vi "Read_Image_Dataset.vi"(4 "Img Width":i32=256, 5 "Norm. Scale":sgl=65535.0, 6 "Img Heigth":i32=256, 7 "Norm. Shift":sgl=65535.0, 8 "error in (no error)":errorcluster, 10 "Annotation file":path, 11 "Image File Paths":path[](array[path])) -> (0 "error out":errorcluster, 3 "Dataset":T1)   [LabVIEW 2020]
uses:
  <vilib>/Ngene/DeepLTK/Toolkit/NN_Data/API/DataSet_Types/NN_DataSet(In3D_Out1D).ctl
  <vilib>/Ngene/DeepLTK/Toolkit/NN_Data/API/DataRef_Types/NN_Data_ref(4D_SGL).ctl
  <vilib>/Ngene/DeepLTK/Toolkit/NN_Data/API/DataRef_Types/NN_Data_ref(2D_SGL).ctl
  <vilib>/Ngene/DeepLTK/Toolkit/NN_Data/Controls/NN_Dims(C,H,W).ctl
  <vilib>/Utility/file.llb/Read Delimited Spreadsheet (string).vi
  <vilib>/vision/NI_Vision_Development_Module.lvlib
  <vilib>/Ngene/DeepLTK/Toolkit/Deep_Learning_Toolkit_by_Ngene.lvlib
panel:
  out "Image Type":T5 items=["Grayscale (U8)", "Grayscale (I16)", "Grayscale (SGL)", "Complex (CSG)", "RGB (U32)", "HSL (U32)", "RGB (U64)", "Grayscale (U16)"]
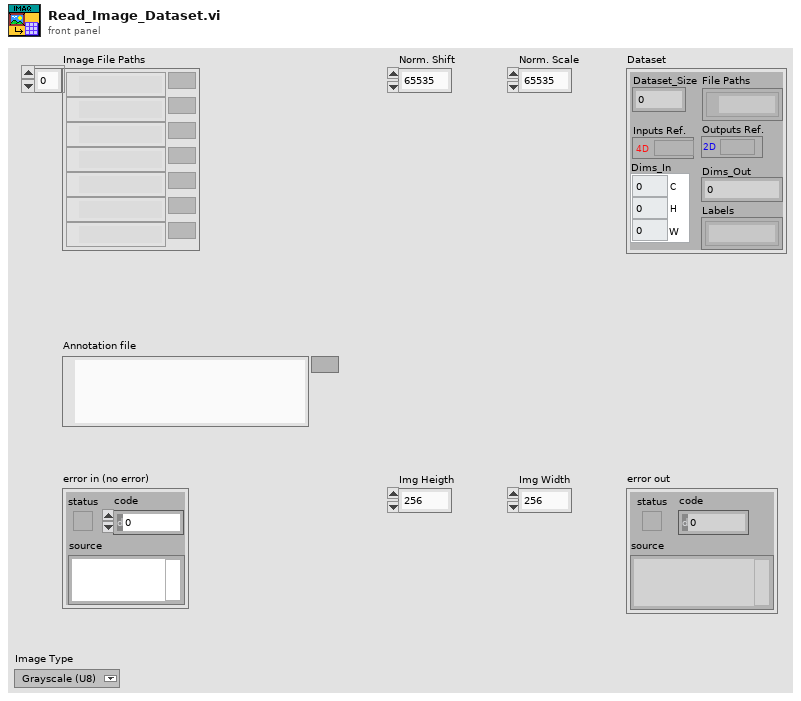
[diagram p1: front panel]
types:
  T1 = typedef "Deep_Learning_Toolkit_by_Ngene.lvlib/NN_DataSet(In3D_Out1D).ctl" = cluster{"Inputs Ref.":T2, "Outputs Ref.":T3, "Dataset_Size":i32, "Dims_In":T4, "Dims_Out":i32, "Labels":string[], "File Paths":path[]}
  T2 = typedef "Deep_Learning_Toolkit_by_Ngene.lvlib/NN_Data_ref(4D_SGL).ctl" = refnum<data-value>
  T3 = typedef "Deep_Learning_Toolkit_by_Ngene.lvlib/NN_Data_ref(2D_SGL).ctl" = refnum<data-value>
  T4 = typedef "Deep_Learning_Toolkit_by_Ngene.lvlib/NN_Dims(C,H,W).ctl" = cluster{"C":i32, "H":i32, "W":i32}
  T5 = typedef "Image Type" = u32
  T6 = typedef "IMAQ Image.ctl" = refnum<image>
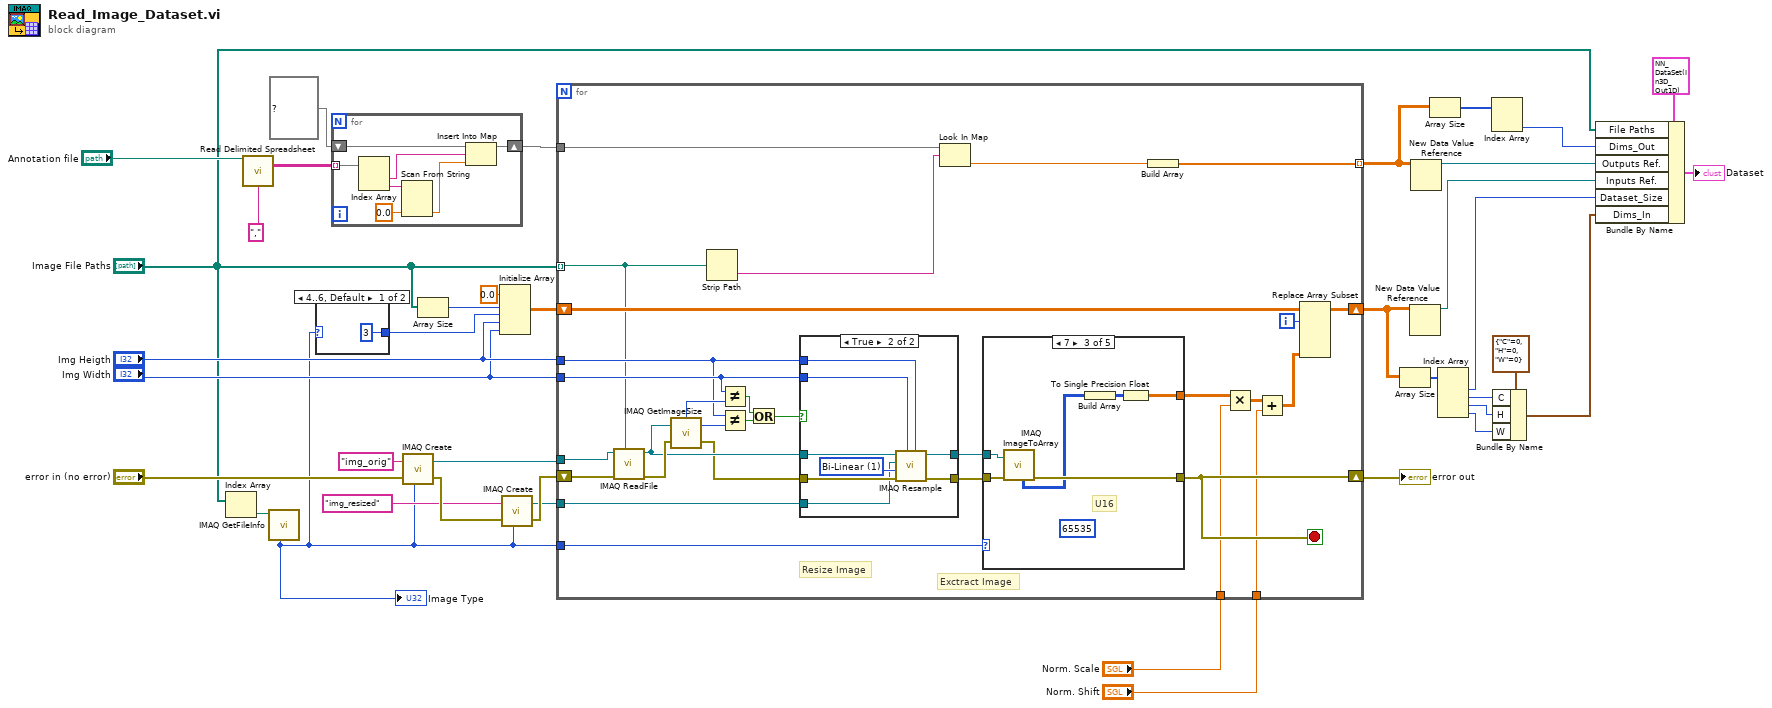
[diagram p0: block diagram]
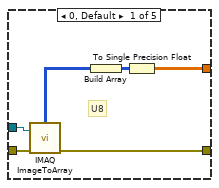
[diagram p2: hidden frame]
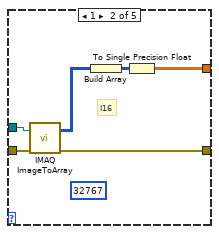
[diagram p3: hidden frame]
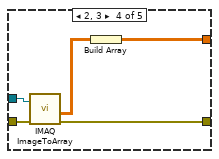
[diagram p4: hidden frame]
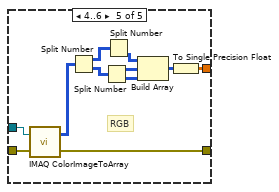
[diagram p5: hidden frame]
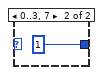
[diagram p7: hidden frame]
diagram:
  n1 = Index Array(array="Image File Paths") -> (element=w26:path)  [unwired: 1 in]
  n2 = call-poly <vilib>:"Read Delimited Spreadsheet.vi"("file path (dialog if empty)"="Annotation file", "delimiter (\\t)"="," ("delimiter (\\t)")) -> ("all rows"=w6:string[][])  [unwired: 8 in, 5 out]
  n3 = call "IMAQ GetFileInfo"("File Path"=w26) -> ("Image Type"=w21:T5)  [unwired: 4 in, 6 out]
  "Image Type" <- w21
  n4 = case shown="4..6, Default" w21 {
    tunnel: [3 ("Chs") 1 ("Chs")] -> w28
    frame 4..6, Default {
    }
    frame 0..3, 7 {
    }
  }
  n5 = for {
    tunnel: w6 -> [w48] mode=indexing
    shift-right: [w43] -> w4
    shift-left: map{string, sgl} {} ("map") -> [w46]
    n6 = Index Array(array=w48) -> (element #1=w45:string, element #2=w47:string)  [unwired: 2 in]
    n7 = Scan From String(input string=w47, default 1=sgl 0.0 ("default value 1")) -> (output 1=w44:sgl)  [unwired: 3 in, 3 out]
    n8 = Insert Into Map(map in=w46, key=w45, value=w44) -> (map out=w43:map{string, sgl})  [unwired: 2 out]
  }
  n9 = call "IMAQ Create"("Image Name"="img_orig", "Image Type"=w21, "error in (no error)"="error in (no error)") -> ("New Image"=w33:T6, "error out"=w39:errorcluster)  [unwired: 2 in]
  n10 = Array Size(array="Image File Paths") -> (size(s)=w18:i32)
  n11 = Initialize Array(sgl 0.0 ("element"), w18, w28, "Img Heigth", "Img Width") -> (w27:sgl[][][][])
  n12 = call "IMAQ Create"("Image Name"="img_resized", "Image Type"=w21, "error in (no error)"=w39) -> ("New Image"=w32:T6, "error out"=w34:errorcluster)  [unwired: 2 in]
  n13 = for {
    tunnel: "Image File Paths" -> [w52] mode=indexing
    tunnel: w33 -> [w78]
    shift-right: [w76] -> w36
    shift-left: w34 -> [w77]
    tunnel: "Img Heigth" -> [w56]
    tunnel: "Img Width" -> [w57]
    tunnel: w32 -> [w65]
    shift-right: [w63] -> w13
    shift-left: w27 -> [w64]
    tunnel: w21 -> [w61]
    tunnel: "Norm. Scale" -> [w55]
    tunnel: "Norm. Shift" -> [w54]
    tunnel: w4 -> [w53]
    tunnel: [w49] -> w2 mode=indexing
    i -> [w62]
    stop <- w76 stop-if-true
    # "Exctract Image"
    # "Resize Image"
    n14 = call "IMAQ ReadFile"("File Path"=w52, "error in (no error)"=w77, "Image"=w78) -> ("error out"=w70:errorcluster, "Image Out"=w69:T6)  [unwired: 4 in, 3 out]
    n15 = call "IMAQ GetImageSize"("Image"=w69, "error in (no error)"=w70) -> ("Y Resolution"=w67:i32, "X Resolution"=w68:i32, "error out"=w66:errorcluster)  [unwired: 2 in]
    n16 = Strip Path(path=w52) -> (name=w51:string)  [unwired: 1 out]
    n17 = Not Equal?(x=w57, y=w68) -> (x != y?=w75:bool)
    n18 = Not Equal?(x=w56, y=w67) -> (x != y?=w71:bool)
    n19 = Or(x=w75, y=w71) -> (x .or. y?=w72:bool)
    n20 = case shown="True" w72 {
      tunnel: [w114 w122] -> w74
      tunnel: w69 -> [w114 w116]
      tunnel: [w113 w121] -> w73
      tunnel: w56 -> [_ w120]
      tunnel: w66 -> [w113 w118]
      tunnel: w57 -> [_ w117]
      tunnel: w65 -> [_ w115]
      frame False {
      }
      frame True {
        w119 = u32 1 items=["Zero Order", "Bi-Linear", "Quadratic", "Cubic Spline"] ("Interpolation Type")
        n21 = call "IMAQ Resample"("X Resolution"=w120, "Y Resolution"=w117, "error in (no error)"=w118, "Interpolation Type"=w119, "Image Dst"=w115, "Image Src"=w116) -> ("error out"=w121:errorcluster, "Image Dst Out"=w122:T6)  [unwired: 4 in]
      }
    }
    n22 = Look In Map(map=w53, key=w51) -> (value=w50:sgl)  [unwired: 1 in, 1 out]
    n23 = case shown="7" w61 {
      tunnel: w74 -> [w80 w87 w93 w99 w106]
      tunnel: w73 -> [w84 w90 w96 w101 w112]
      tunnel: [w82 w89 w95 w100 w110] -> w76
      tunnel: [w79 w86 w92 w98 w102] -> w59
      frame 0, Default {
        # "U8"
        n24 = call "IMAQ ImageToArray"("error in (no error)"=w84, "Image"=w80) -> ("error out"=w82:errorcluster, "Image Pixels (U8)"=w83:u8[][])  [unwired: 2 in, 3 out]
        n25 = Build Array(w83) -> (w81:u8[][][])
        n26 = To Single Precision Float(number=w81) -> (single precision float=w79:sgl[][][])
      }
      frame 1 {
        (unwired) i16 32767
        # "I16"
        n27 = call "IMAQ ImageToArray"("error in (no error)"=w90, "Image"=w87) -> ("error out"=w89:errorcluster, "Image Pixels (I16)"=w85:i16[][])  [unwired: 2 in, 3 out]
        n28 = Build Array(w85) -> (w88:i16[][][])
        n29 = To Single Precision Float(number=w88) -> (single precision float=w86:sgl[][][])
      }
      frame 7 {
        (unwired) u16 65535
        # "U16"
        n30 = call "IMAQ ImageToArray"("error in (no error)"=w96, "Image"=w93) -> ("Image Pixels (U16)"=w91:u16[][], "error out"=w95:errorcluster)  [unwired: 2 in, 3 out]
        n31 = Build Array(w91) -> (w94:u16[][][])
        n32 = To Single Precision Float(number=w94) -> (single precision float=w92:sgl[][][])
      }
      frame 2, 3 {
        n33 = call "IMAQ ImageToArray"("error in (no error)"=w101, "Image"=w99) -> ("Image Pixels (Float)"=w97:sgl[][], "error out"=w100:errorcluster)  [unwired: 2 in, 3 out]
        n34 = Build Array(w97) -> (w98:sgl[][][])
      }
      frame 4..6 {
        # "RGB"
        n35 = call "IMAQ ColorImageToArray"("Image"=w106, "error in (no error)"=w112) -> ("Image Pixels (U32)"=w111:u32[][], "error out"=w110:errorcluster)  [unwired: 2 in, 1 out]
        n36 = Split Number(x=w111) -> (hi(x)=w108:u16[][], lo(x)=w109:u16[][])
        n37 = Split Number(x=w109) -> (hi(x)=w104:u8[][], lo(x)=w103:u8[][])
        n38 = Split Number(x=w108) -> (lo(x)=w105:u8[][])  [unwired: 1 out]
        n39 = Build Array(w105, w104, w103) -> (w107:u8[][][])
        n40 = To Single Precision Float(number=w107) -> (single precision float=w102:sgl[][][])
      }
    }
    n41 = Build Array(w50) -> (w49:sgl[])
    n42 = Multiply(x=w59, y=w55) -> (x*y=w60:sgl[][][])
    n43 = Add(x=w60, y=w54) -> (x+y=w58:sgl[][][])
    n44 = Replace Array Subset(array=w64, new element=w58, index (dim 0)=w62) -> (w63:sgl[][][][])  [unwired: 3 in]
  }
  "error out" <- w36
  n45 = Array Size(array=w13) -> (size(s)=w25:i32[])
  n46 = New Data Value Reference(data value=w13) -> (data value reference=w12:refnum<data-value>)  [unwired: 1 in, 1 out]
  n47 = New Data Value Reference(data value=w2) -> (data value reference=w11:refnum<data-value>)  [unwired: 1 in, 1 out]
  n48 = Array Size(array=w2) -> (size(s)=w17:i32[])
  n49 = Index Array(array=w25) -> (element #1=w10:i32, element #2=w24:i32, element #3=w23:i32, element #4=w22:i32)  [unwired: 4 in]
  n50 = Index Array(array=w17) -> (element #2=w1:i32)  [unwired: 2 in, 1 out]
  n51 = Bundle By Name(cluster=T4 {"C"=0, "H"=0, "W"=0} ("Dims(C,H,W)"), "C"=w24, "H"=w23, "W"=w22) -> (w9:T4)
  n52 = Bundle By Name(cluster=T1 {"Inputs Ref."=refnum, "Outputs Ref."=refnum, "Dataset_Size"=0, "Dims_In"={"C"=0, "H"=0, "W"=0}, "Dims_Out"=0, "Labels"=[], "File Paths"=[]} ("Dataset Refs. (In3D_Out1D)"), "File Paths"="Image File Paths", "Dims_Out"=w1, "Outputs Ref."=w11, "Inputs Ref."=w12, "Dataset_Size"=w10, "Dims_In"=w9) -> (→"Dataset":T1)
